vi "Validate Loopback Channels.vi"(6 "index":i32, 8 "error in (no error)":errorcluster, 9 "additional channel values to write":dbl[](array[numeric]), 10 "channels":T1, 11 "CAN Loopback Tests in":refnum<class "CAN Loopback Tests.lvclass">) -> (0 "error out":errorcluster, 1 "additional channel values to read":dbl[](array[numeric]), 2 "loopback channel values to read":dbl[](array[numeric]), 3 "CAN Loopback Tests out":refnum<class "CAN Loopback Tests.lvclass">)   [LabVIEW 2017, in "CAN Loopback Tests.lvclass"]
uses:
  CAN Loopback Tests.lvclass
  C:/Users/nitest/Documents/ni-official/niveristand-custom-device-testing-tools/VeriStandTestCase/VeriStandTestCase.lvclass
  2322e7bb-a155-470f-b43d-e4e34841ee51.vi
  <vilib>/NI Veristand/Execution/Workspace/NI VeriStand - Set Multiple Channel Values.vi
  <vilib>/NI Veristand/Execution/Workspace/NI VeriStand - Get Multiple Channel Values.vi
  <vilib>/NI VeriStand/Execution/Workspace/NI_VS Workspace ExecutionAPI.lvlib
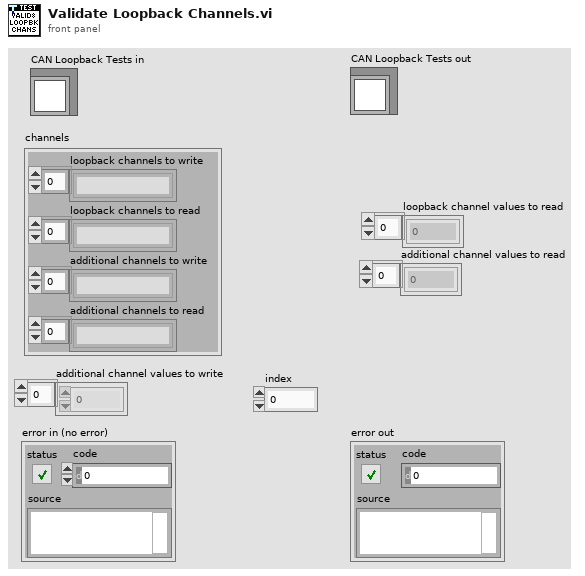
[diagram p1: front panel]
types:
  T1 = cluster{"loopback channels to write":string[], "loopback channels to read":string[], "additional channels to write":string[], "additional channels to read":string[]}
  T2 = typedef "NI_VS Workspace ExecutionAPI.lvlib/WorkspaceAPI.ctl" = refnum<k24>
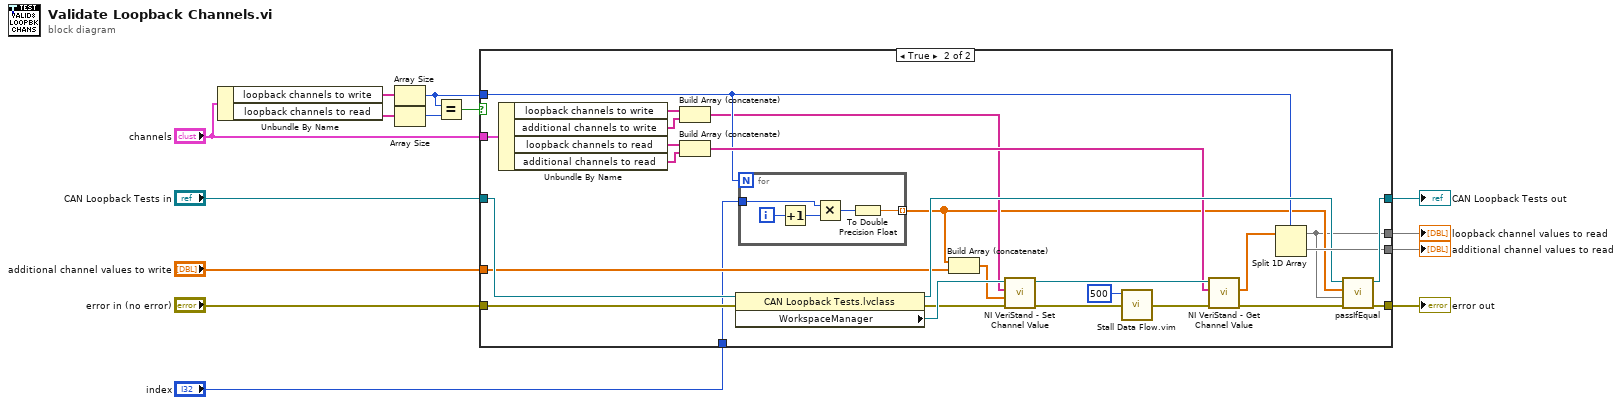
[diagram p0: block diagram]
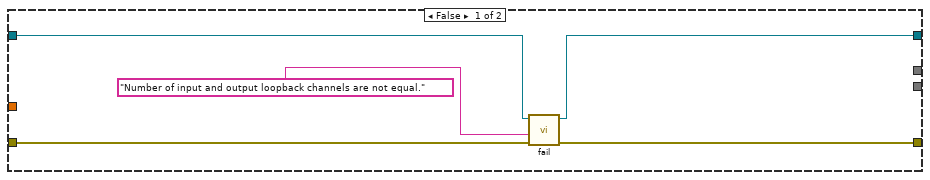
[diagram p2: hidden frame]
diagram:
  n1 = Unbundle By Name("channels") -> ("loopback channels to write"=w9:string[], "loopback channels to read"=w8:string[])
  n2 = Array Size(array=w9) -> (size(s)=w4:i32)
  n3 = Array Size(array=w8) -> (size(s)=w5:i32)
  n4 = Equal?(x=w4, y=w5) -> (x = y?=w10:bool)
  n5 = case shown="True" w10 {
    tunnel: [w17 w46] -> w14
    tunnel: [_ w45] -> w6
    tunnel: [w18 w43] -> w13
    tunnel: "CAN Loopback Tests in" -> [w16 w36]
    tunnel: "error in (no error)" -> [w19 w34]
    tunnel: w4 -> [_ w29]
    tunnel: "channels" -> [_ w30]
    tunnel: "additional channel values to write" -> [_ w22]
    tunnel: "index" -> [_ w20]
    tunnel: [_ w21] -> w1
    frame False {
      n6 = call-dynamic "fail.vi"("error in (no error)"=w19, "message (\"\")"="Number of input and output loopback channels are not equal." ("message (\"\")"), "TestCase in"=w16) -> ("error out"=w18:errorcluster, "TestCase out"=w17:refnum<class "CAN Loopback Tests.lvclass">)  [unwired: 7 in]
    }
    frame True {
      n7 = Unbundle By Name(w30) -> ("loopback channels to write"=w27:string[], "additional channels to write"=w25:string[], "loopback channels to read"=w28:string[], "additional channels to read"=w32:string[])
      n8 = Build Array (concatenate)(w27, w25) -> (w26:string[])
      n9 = Build Array (concatenate)(w28, w32) -> (w31:string[])
      n10 = property class="CAN Loopback Tests.lvclass"(reference=w36, error in=w34) -> (reference out=w35:refnum<class "CAN Loopback Tests.lvclass">, error out=w33:errorcluster, "WorkspaceManager"=w37:T2)
      n11 = for {
        N: w29 -> [_]
        tunnel: [w47] -> w23 mode=indexing
        tunnel: w20 -> [w51]
        i -> [w50]
        n12 = Increment(x=w50) -> (x+1=w48:i32)
        n13 = Multiply(x=w51, y=w48) -> (x*y=w49:i32)
        n14 = To Double Precision Float(number=w49) -> (double precision float=w47:dbl)
      }
      n15 = Build Array (concatenate)(w23, w22) -> (w24:dbl[])
      n16 = call-poly <vilib>:"NI VeriStand - Set Channel Value.vi"("error in (no error)"=w33, "Values"=w24, "Channels"=w26, "WorkspaceManager in"=w37) -> ("error out"=w38:errorcluster, "WorkspaceManager out"=w42:T2)  [unwired: 6 in]
      n17 = call "Stall Data Flow.vim"("value in"=w38, "milliseconds to wait"=u32 500) -> ("value out"=w39:errorcluster)  [unwired: 1 out]
      n18 = call-poly <vilib>:"NI VeriStand - Get Channel Value.vi"("error in (no error)"=w39, "Channels"=w31, "WorkspaceManager in"=w42) -> ("error out"=w40:errorcluster, "Values"=w44:dbl[])  [unwired: 6 in, 1 out]
      n19 = Split 1D Array(array=w44, index=w29) -> (first subarray=w21:dbl[], second subarray=w45:dbl[])
      n20 = call-dynamic "passIfEqual.vi"("error in (no error)"=w40, "y"=w21, "x"=w23, "TestCase in"=w35) -> ("error out"=w43:errorcluster, "TestCase out"=w46:refnum<class "CAN Loopback Tests.lvclass">)  [unwired: 6 in]
    }
  }
  "CAN Loopback Tests out" <- w14
  "error out" <- w13
  "additional channel values to read" <- w6
  "loopback channel values to read" <- w1
